vi "Save Settings to XML.vi"(8 "error in (no error)":errorcluster, 11 "Settings":T1={"Hardware Configuration"={"DAQmx Task"="", "Counter(s)"="Dev2/ctr0", "samples per readout"=0}, "Logging Configuration"={"Log File Base Path"=path "", "Max Samples"=0, "File Refnum"=refnum, "Log Piezo"=FALSE, "Piezo File Refnum"=refnum}, "Piezo Config"={"Piezo Serial Number"=41848555, "MG17Piezo"=refnum, "Setpoint (um)"=0.0}, "Capacitive Config"={"IP Address"="192.168.168.57", "Handle"=0, "Refresh Time (ms)"=0.0}}) -> (0 "error out":errorcluster)   [LabVIEW 2013, in "Settings.lvlib"]
doc: "Saves the \"User Specified\" configuration data to an XML file. This is used to remember the users settings between executions."
uses:
  Settings.lvlib
  Settings.ctl
  Acquisition/Hardware Configuration.ctl
  Logging/Logging Configuration.ctl
  Piezo/Hardware Configuration.ctl
  Capacitive/Hardware Configuration.ctl
  <vilib>/Utility/xml.llb/Write to XML File(string).vi
  Acquisition/Acquisition.lvlib
  Logging/Logging.lvlib
  Desktop/Simon Labview/Piezo.lvlib
  Capacitive/Capacitive.lvlib
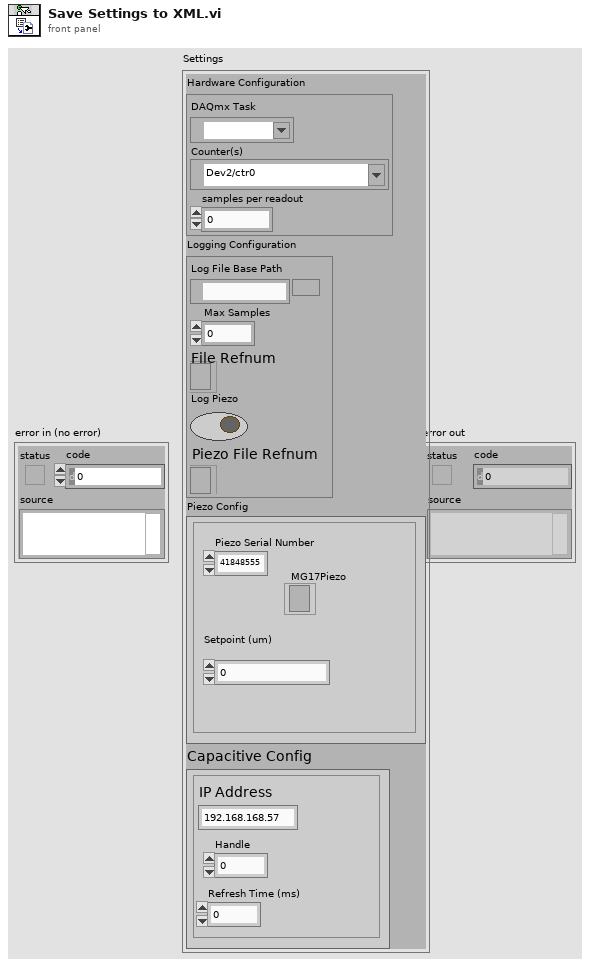
[diagram p1: front panel]
types:
  T1 = typedef "Settings.lvlib/Settings.ctl" = cluster{"Hardware Configuration":T2, "Logging Configuration":T3, "Piezo Config":T4, "Capacitive Config":T5}
  T2 = typedef "Acquisition.lvlib/Hardware Configuration.ctl" = cluster{"DAQmx Task":refnum<k21>, "Counter(s)":tag, "samples per readout":i32}
  T3 = typedef "Logging.lvlib/Logging Configuration.ctl" = cluster{"Log File Base Path":path, "Max Samples":u32, "File Refnum":refnum<file>, "Log Piezo":bool, "Piezo File Refnum":refnum<file>}
  T4 = typedef "Piezo.lvlib/Hardware Configuration.ctl" = cluster{"Piezo Serial Number":i32, "MG17Piezo":refnum<k7>, "Setpoint (um)":sgl}
  T5 = typedef "Capacitive.lvlib/Hardware Configuration.ctl" = cluster{"IP Address":string, "Handle":u32, "Refresh Time (ms)":dbl}
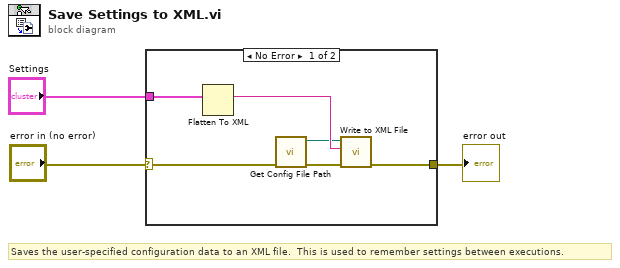
[diagram p0: block diagram]
diagram:
  # "Saves the user-specified configuration data to an XML file.  This is used to remember settings between executions."
  n1 = case shown="No Error" "error in (no error)" {
    selector: "error in (no error)" -> [w5 w10]
    tunnel: [w7 w10] -> w2
    tunnel: "Settings" -> [w9 _]
    frame No Error {
      n2 = Flatten To XML(anything=w9) -> (xml string=w8:string)
      n3 = call "Get Config File Path.vi"("error in (no error)"=w5) -> ("error out"=w4:errorcluster, "XML File Path"=w6:path)  [unwired: 9 in]
      n4 = call-poly <vilib>:"Write to XML File.vi"("error in (no error)"=w4, "XML Input"=w8, "XML File Path"=w6) -> ("error out"=w7:errorcluster)  [unwired: 6 in, 2 out]
    }
    frame Error {
    }
  }
  "error out" <- w2
